vi "Empty Message Queues.vi"(8 "error out":errorcluster, 11 "dup Message Queue":refnum<queue>) -> (0 "error out 2":errorcluster)   [LabVIEW 2019]
uses:
  Message Cluster.ctl
  Message Queue.lvlib
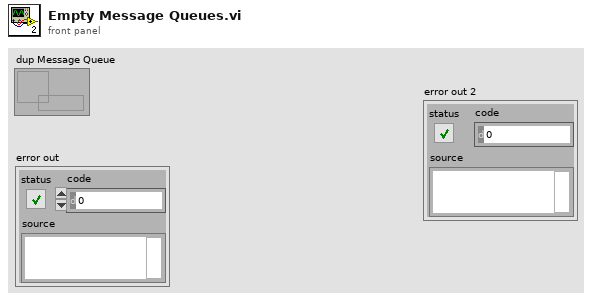
[diagram p1: front panel]
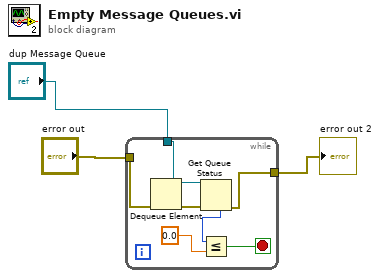
[diagram p0: block diagram]
diagram:
  n1 = while {
    tunnel: "dup Message Queue" -> [w10]
    tunnel: "error out" -> [w11]
    tunnel: [w4] -> w2
    stop <- w5 stop-if-true
    n2 = Dequeue Element(queue=w10, error in (no error)=w11) -> (queue out=w8:refnum<queue>, error out=w9:errorcluster)  [unwired: 1 in, 2 out]
    n3 = Get Queue Status(queue=w8, error in (no error)=w9) -> (error out=w4:errorcluster, # elements in queue=w6:i32)  [unwired: 1 in, 6 out]
    n4 = Less Or Equal?(x=w6, y=0.0) -> (x <= y?=w5:bool)
  }
  "error out 2" <- w2
